vi "GET HTTP.vi"(8 "error in (no error)":errorcluster, 10 "URL":string, 11 "output file":path) -> (0 "error out":errorcluster)   [LabVIEW 2021, in "lv_IconEditor.lvlib"]
uses:
  <resource>/plugins/lv_IconEditor.lvlib
  <vilib>/Utility/error.llb/Trim Whitespace One-Sided.vi
  <vilib>/httpClient/LabVIEWHTTPClient.lvlib
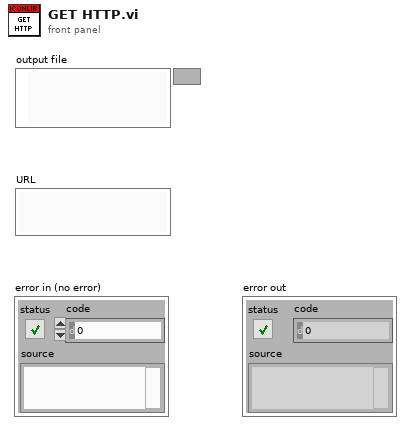
[diagram p1: front panel]
types:
  T1 = typedef "LabVIEWHTTPClient.lvlib/ClientHandle.ctl" = refnum<k1>
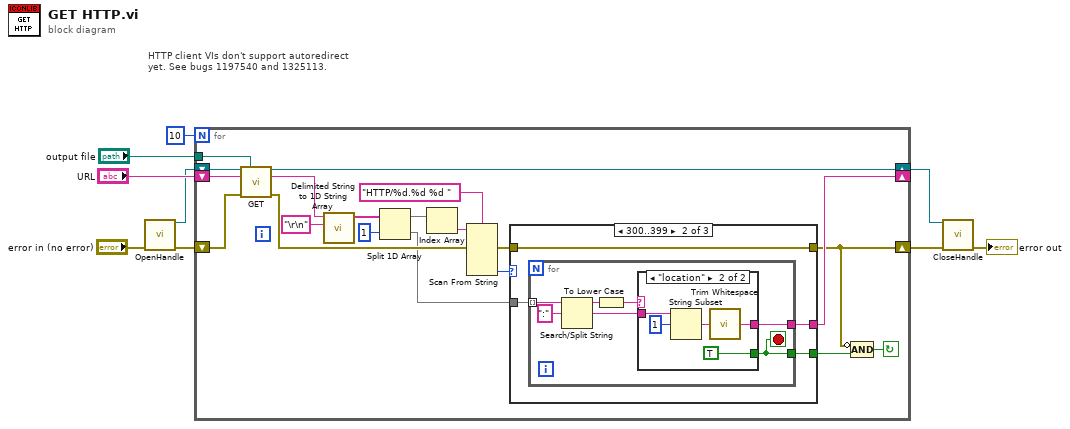
[diagram p0: block diagram]
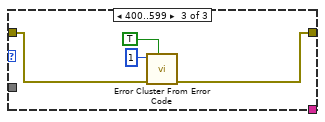
[diagram p4: hidden frame]
diagram:
  # "HTTP client VIs don't support autoredirect yet. See bugs 1197540 and 1325113."
  n1 = call <vilib>:"OpenHandle.vi"("error in (no error)"="error in (no error)") -> ("client handle out"=w4:T1, "error out"=w5:errorcluster)  [unwired: 13 in]
  n2 = for {
    N: 10 -> [_]
    tunnel: "output file" -> [w26]
    shift-right: [w28] -> w1
    shift-left: w4 -> [w29]
    shift-right: [w10] -> w3
    shift-left: w5 -> [w27]
    shift-right: [w21] -> _
    shift-left: "URL" -> [w25]
    stop <- w23 continue-if-true
    n3 = call <vilib>:"GET.vi"("client handle"=w29, "output file"=w26, "url"=w25, "error in (no error)"=w27) -> ("client handle out"=w28:T1, "headers"=w20:string, "error out"=w22:errorcluster)  [unwired: 8 in, 1 out]
    n4 = call <vilib>:"Delimited String to 1D String Array.vi"("delimiter"="\r\n", "delimited string"=w20) -> ("string array"=w15:string[])  [unwired: 9 in]
    n5 = Split 1D Array(array=w15, index=1) -> (first subarray=w17:string[], second subarray=w18:string[])
    n6 = Index Array(array=w17) -> (element=w13:string)  [unwired: 1 in]
    n7 = Scan From String(format string="HTTP/%d.%d %d ", input string=w13, error in=w22) -> (error out=w11:errorcluster, output 3=w19:i32)  [unwired: 6 in, 2 out]
    n8 = case shown="300..399" w19 {
      tunnel: w18 -> [_ w34 _]
      tunnel: [_ w33 _] -> w21
      tunnel: [_ w32 _] -> w24
      tunnel: w11 -> [w30 w31 w48]
      tunnel: [w30 w31 w47] -> w10
      frame Default {
      }
      frame 300..399 {
        n9 = for {
          tunnel: w34 -> [w41] mode=indexing
          tunnel: [w36] -> w33
          tunnel: [w35] -> w32
          stop <- w35 stop-if-true
          n10 = Search/Split String(string=w41, search string/char (-)=":") -> (substring before match=w38:string, match + rest of string=w39:string)  [unwired: 1 in, 1 out]
          n11 = To Lower Case(string=w38) -> (all lower case string=w37:string)
          n12 = case shown="\"location\"" w37 {
            tunnel: w39 -> [_ w46]
            tunnel: [_ w43] -> w36
            tunnel: [_ TRUE] -> w35
            frame Default {
            }
            frame "location" {
              n13 = String Subset(string=w46, offset (0)=1) -> (substring=w44:string)  [unwired: 1 in]
              n14 = call <vilib>:"Trim Whitespace.vi"("string"=w44) -> ("trimmed string"=w43:string)  [unwired: 1 in]
            }
          }
        }
      }
      frame 400..599 {
        n15 = call <vilib>:"Error Cluster From Error Code.vi"("show call chain? (False)"=TRUE, "error in (no error)"=w48, "error code (0)"=1) -> ("error out"=w47:errorcluster)  [unwired: 6 in]
      }
    }
    n16 = Compound Arithmetic op=AND(invert w10, w24) -> (w23:bool)
  }
  n17 = call <vilib>:"CloseHandle.vi"("client handle"=w1, "error in (no error)"=w3) -> ("error out"=→"error out":errorcluster)  [unwired: 13 in]
